vi "Report CH Name to Number.vi"(11 "Ch Name":string="Card2 Ch 4") -> (3 "Ch number":i32)   [LabVIEW 2020]
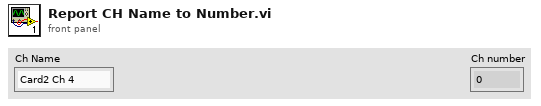
[diagram p1: front panel]
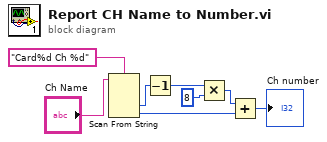
[diagram p0: block diagram]
diagram:
  n1 = Scan From String(format string="Card%d Ch %d", input string="Ch Name") -> (output 1=w6:i32, output 2=w3:i32)  [unwired: 4 in, 3 out]
  n2 = Decrement(x=w6) -> (x-1=w1:i32)
  n3 = Multiply(x=w1, y=8) -> (x*y=w4:i32)
  n4 = Add(x=w4, y=w3) -> (x+y=→"Ch number":i32)
